vi "create_text_message.vi"(8 "error in (no error)":errorcluster, 10 "content":string[](array[string]), 11 "role":string) -> (0 "error out":errorcluster, 3 "message_text out":refnum<class "message_text.lvclass">)   [LabVIEW 2020, in "message_text.lvclass"]
uses:
  message_text.lvclass
  message.ctl
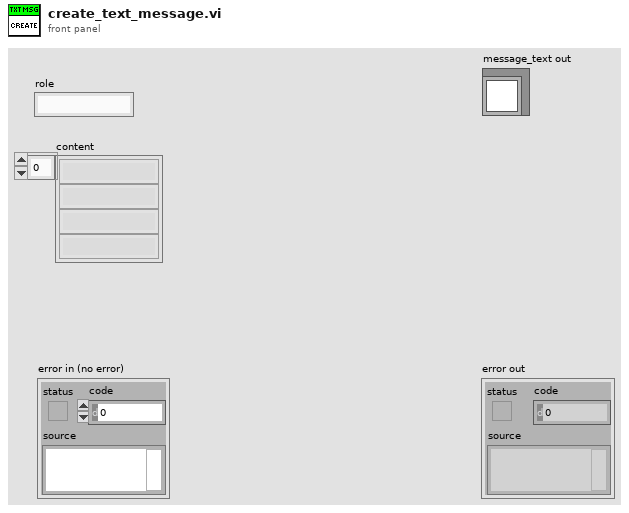
[diagram p1: front panel]
types:
  T1 = typedef "message_text.lvclass/message.ctl" = cluster{"role":string, "content":string[]}
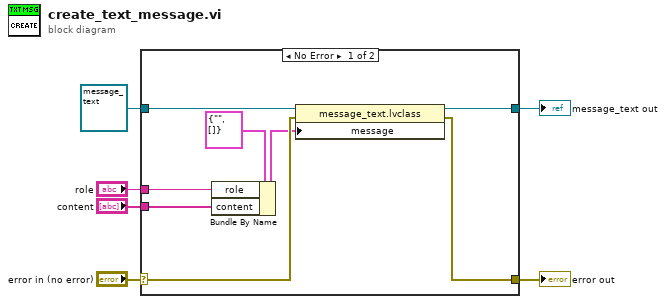
[diagram p0: block diagram]
diagram:
  n1 = case shown="No Error" "error in (no error)" {
    selector: "error in (no error)" -> [w12 w16]
    tunnel: [w11 w16] -> w5
    tunnel: [w13 w15] -> w3
    tunnel: refnum<class "message_text.lvclass"> refnum ("message_text in") -> [w14 w15]
    tunnel: "content" -> [w8 _]
    tunnel: "role" -> [w7 _]
    frame No Error {
      n2 = Bundle By Name(cluster=T1 {"role"="", "content"=[]} ("message"), "role"=w7, "content"=w8) -> (w9:T1)
      n3 = property class="message_text.lvclass"(reference=w14, error in=w12, "message"=w9) -> (reference out=w13:refnum<class "message_text.lvclass">, error out=w11:errorcluster)
    }
    frame Error {
    }
  }
  "error out" <- w5
  "message_text out" <- w3
